vi "Least square fit uncertainties.vi"(9 "Best Linear Fit":dbl[](array[numeric])=[-82227.49073478492, -79428.81430499739, -76720.52498891533, -74343.19475156673, -71953.92816409204, -69899.28508654764, -68651.42427883964, -65998.20719202016, -63062.026560482176, -58952.42528894555, -55664.08709951259], 10 "Y":dbl[](array[numeric])=[-82394.3661971831, -79859.15492957746, -77323.94366197183, -74788.73239436619, -72253.52112676056, -69718.30985915492, -67183.0985915493, -64647.88732394366, -62112.67605633802, -59577.464788732395, -57042.25352112676], 11 "X":dbl[](array[numeric])=[0.004563028395882726, 0.004381964238647146, 0.004206747797994251, 0.0040529432026095435, 0.0038983663689078074, 0.0037654384558072074, 0.0036847064129421764, 0.003513052944654496, 0.003323092767092556, 0.0030572165540065227, 0.0028444730668930607]) -> (0 "sigma_B (Oe/V)":dbl=553586.18151728, 3 "sigma_A (Oe)":dbl=2097.5321873084963)   [LabVIEW 2013]
panel:
  # "Uncertainties in A and B\ny=A+Bx"
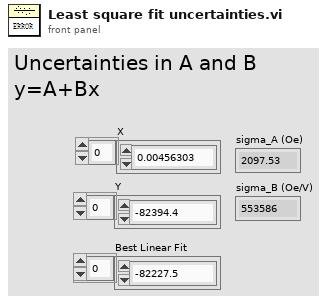
[diagram p1: front panel]
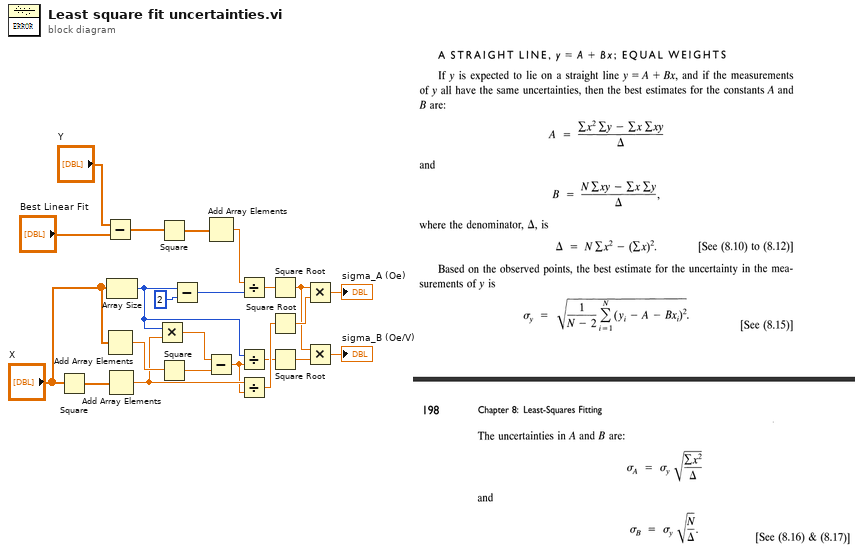
[diagram p0: block diagram]
diagram:
  n1 = Square(x="X") -> (x^2=w11:dbl[])
  n2 = Subtract(x="Y", y="Best Linear Fit") -> (x-y=w20:dbl[])
  n3 = Add Array Elements(numeric array="X") -> (sum=w14:dbl)
  n4 = Add Array Elements(numeric array=w11) -> (sum=w8:dbl)
  n5 = Array Size(array="X") -> (size(s)=w6:i32)
  n6 = Multiply(x=w6, y=w8) -> (x*y=w13:dbl)
  n7 = Square(x=w20) -> (x^2=w19:dbl[])
  n8 = Square(x=w14) -> (x^2=w12:dbl)
  n9 = Subtract(x=w6, y=2) -> (x-y=w17:i32)
  n10 = Add Array Elements(numeric array=w19) -> (sum=w18:dbl)
  n11 = Subtract(x=w13, y=w12) -> (x-y=w5:dbl)
  n12 = Divide(x=w18, y=w17) -> (x/y=w16:dbl)
  n13 = Divide(x=w6, y=w5) -> (x/y=w4:dbl)
  n14 = Divide(x=w8, y=w5) -> (x/y=w10:dbl)
  n15 = Square Root(x=w16) -> (sqrt(x)=w3:dbl)
  n16 = Square Root(x=w10) -> (sqrt(x)=w9:dbl)
  n17 = Square Root(x=w4) -> (sqrt(x)=w2:dbl)
  n18 = Multiply(x=w3, y=w9) -> (x*y=→"sigma_A (Oe)":dbl)
  n19 = Multiply(x=w3, y=w2) -> (x*y=→"sigma_B (Oe/V)":dbl)
